vi "Call Easing Function Dynamically.vi"(8 "error in":errorcluster, 11 "Display State In":T1={"Numeric"=0.0, "Array of Button References"=[], "Space Between Menu Buttons"=0, "Number of Menu Buttons"=0, "Array of Button Names"=[], "Most Recent Vertical Position"=0, "This VI"=refnum, "Current Action"=enum."Not Moving", "Most Recent Distance Traveled"=0, "Method"=enum."Move Up", "Data In"=0} caption="State") -> (0 "error out":errorcluster, 3 "Display State Out":T1={"Numeric"=0.0, "Array of Button References"=[], "Space Between Menu Buttons"=0, "Number of Menu Buttons"=0, "Array of Button Names"=[], "Most Recent Vertical Position"=0, "This VI"=refnum, "Current Action"=enum."Not Moving", "Most Recent Distance Traveled"=0, "Method"=enum."Move Up", "Data In"=0} caption="State")   [LabVIEW 2011, in "Sliding Menu Library.lvlib" / "Sliding Menu XControl.xctl"]
uses:
  Sliding Menu XControl.xctl
  Sliding Menu State.ctl
  Menu Button Library/Menu Button xControl/Menu Button xControl.xctl
  Sliding Menu SubVIs/Sliding Menu Type Definitions/Current User Action.ctl
  Sliding Menu Methods.ctl
  Sliding Menu Data.ctl
  Sliding Menu Library.lvlib
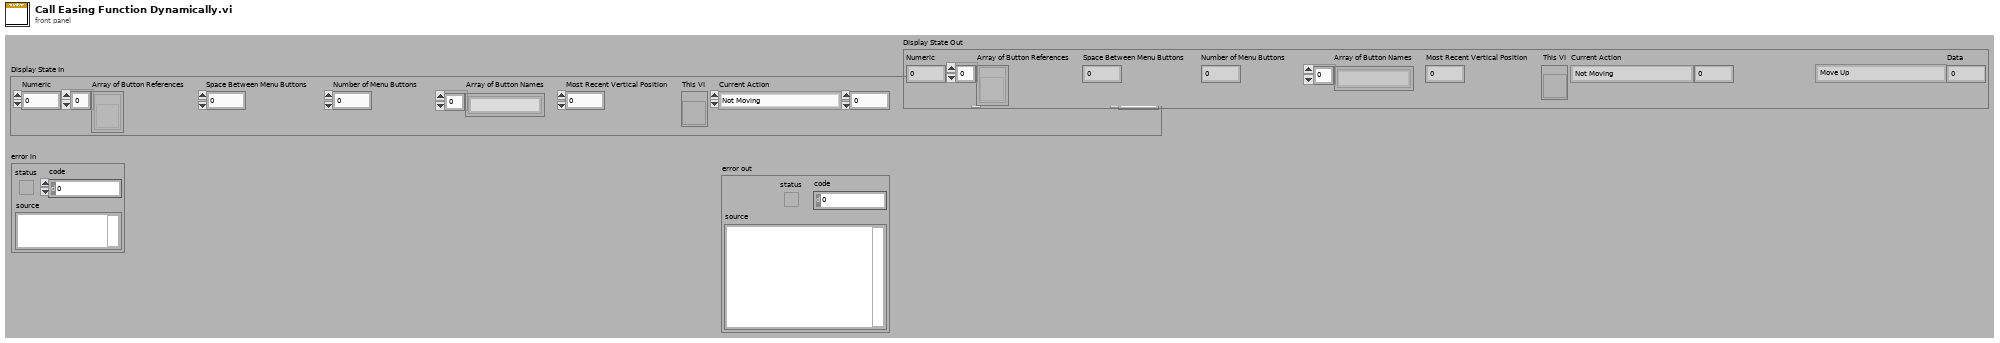
[diagram p1: front panel]
types:
  T1 = typedef "Sliding Menu Library.lvlib/Sliding Menu XControl.xctl/Sliding Menu State.ctl" = cluster{"Numeric":dbl, "Array of Button References":refnum<vi>[], "Space Between Menu Buttons":i32, "Number of Menu Buttons":i32, "Array of Button Names":string[], "Most Recent Vertical Position":i32, "This VI":refnum<vi>, "Current Action":T2, "Most Recent Distance Traveled":i32, "Method":T3, "Data In":T4}
  T2 = typedef "Sliding Menu Library.lvlib/Current User Action.ctl" = enum16{"Not Moving", "Mouse Down", "Mouse Up No Dragging", "Bounce Up Needed", "Bounce Down Needed", "Dragging", "Easing"}
  T3 = typedef "Sliding Menu Methods.ctl" = enum16{"Resize", "Move Up", "Move Down", "Move to 0"}
  T4 = typedef "Sliding Menu Library.lvlib/Sliding Menu XControl.xctl/Sliding Menu Data.ctl" = i32
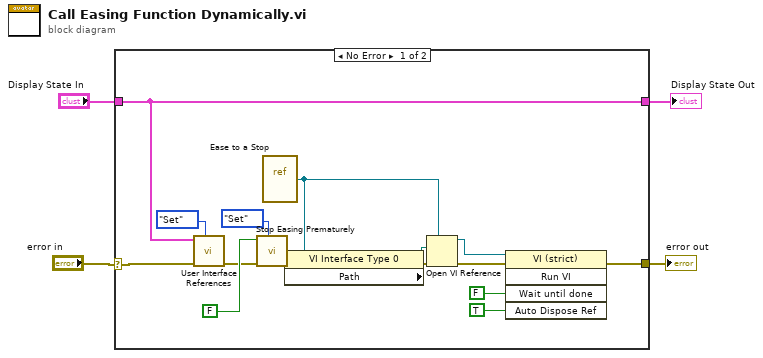
[diagram p0: block diagram]
diagram:
  n1 = case shown="No Error" "error in" {
    selector: "error in" -> [w6 w20]
    tunnel: [w14 w20] -> w4
    tunnel: "Display State In" -> [w5 w21]
    tunnel: [w5 w21] -> w1
    frame No Error {
      n2 = call "User Interface References.vi"("Set or Get Value"=enum16{"Set", "Get"}."Set", "error in"=w6, "Display State In"=w5) -> ("error out"=w8:errorcluster)  [unwired: 7 in, 1 out]
      n3 = call "Stop Easing Prematurely.vi"("Set or Get Value"=enum16{"Set", "Get"}."Set", "error in"=w8, "Stop?"=FALSE) -> ("error out"=w7:errorcluster)  [unwired: 7 in, 1 out]
      n4 = vi-ref "Ease to a Stop.vi"() -> (w18:refnum<vi>)
      n5 = property class="VI Interface Type 0"(reference=w18, error in=w7) -> (error out=w19:errorcluster, "Path"=w17:path)  [unwired: 1 out]
      n6 = Open VI Reference(type specifier VI Refnum (for type only)=w18, vi path=w17, error in (no error)=w19) -> (vi reference=w13:refnum<vi>, error out=w12:errorcluster)  [unwired: 3 in]
      n7 = invoke class="VI (strict)" method="Run VI"(reference=w13, error in=w12, "Wait until done"=FALSE ("Wait Until Done"), "Auto Dispose Ref"=TRUE ("Auto Dispose Reference")) -> (error out=w14:errorcluster)  [unwired: 1 in, 4 out]
    }
    frame Error {
    }
  }
  "error out" <- w4
  "Display State Out" <- w1
